vi "Empty Syringe.vi"(8 "error in (no error)":errorcluster, 9 "auto_switch_valve":bool=TRUE, 10 "flow_rate_uL_s":dbl=400.0) -> (0 "error out":errorcluster)   [LabVIEW 2018, in "cetoni.lvlib" / "cetoni.lvclass"]
uses:
  cetoni.lvclass
  <userlib>/QmixLib/QmixLib.lvlib
  Program Files/cetoni/QmixSDK/lib/labview/labbCAN_Pump_API/labbCAN_Pump_API.lvlib
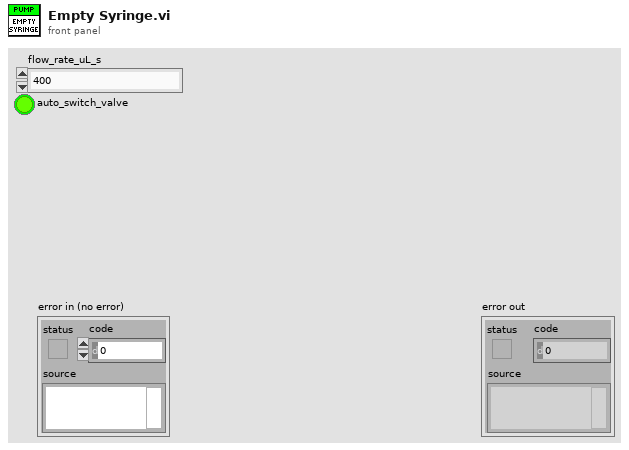
[diagram p1: front panel]
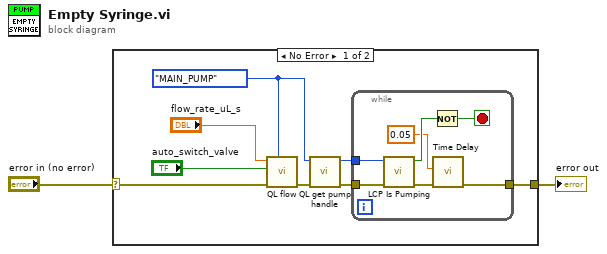
[diagram p0: block diagram]
diagram:
  n1 = case shown="No Error" "error in (no error)" {
    selector: "error in (no error)" -> [w10 w18]
    tunnel: [w8 w18] -> w1
    frame No Error {
      w5 = enum16{"MAIN_PUMP"}."MAIN_PUMP" ("pump")
      n2 = call <userlib>:"QL flow.vi"("pump"=w5, "error in (no error)"=w10, "auto_switch_valve"="auto_switch_valve", "flow_rate_uL_s"="flow_rate_uL_s") -> ("error out"=w7:errorcluster)  [unwired: 7 in]
      n3 = call <userlib>:"QL get pump handle.vi"("error in (no error)"=w7, "pump"=w5) -> ("error out"=w6:errorcluster, "pump handle"=w4:u64)  [unwired: 8 in]
      n4 = while {
        tunnel: w6 -> [w12]
        tunnel: [w14] -> w8
        tunnel: w4 -> [w11]
        stop <- w17 stop-if-true
        n5 = call "LCP Is Pumping.vi"("error in (no error)"=w12, "Pump Handle"=w11) -> ("error out"=w15:errorcluster, "Is pumping"=w16:bool)  [unwired: 8 in]
        n6 = Not(x=w16) -> (.not. x?=w17:bool)
        n7 = call "Time Delay"("error in (no error)"=w15, "Delay Time (s)"=0.05) -> ("error out"=w14:errorcluster)  [unwired: 9 in]
      }
    }
    frame Error {
    }
  }
  "error out" <- w1
